vi "Shrug Pipette.vi"(4 "Pressure Controls":T1, 6 "Pressure Levels":refnum<vi>, 8 "error in (no error)":errorcluster, 10 "Manipulator Dynamics":refnum<vi>, 11 "VISA resource in":refnum<visa-resource-name>="COM1") -> (0 "error out":errorcluster, 3 "VISA resource out":refnum<visa-resource-name>)   [LabVIEW 2012, in "Autopatcher Daemon.lvlib"]
uses:
  Autopatcher Daemon.lvlib
  Scientifica Manipulator Controls.lvlib
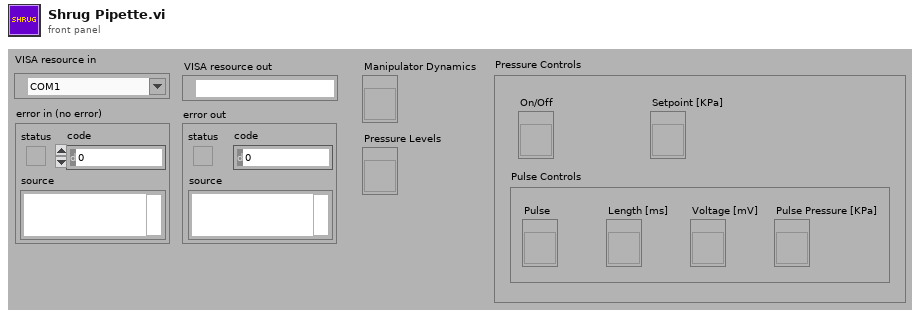
[diagram p1: front panel]
types:
  T1 = cluster{"Setpoint [KPa]":refnum<vi>, "On/Off":refnum<vi>, "Pulse Controls":cluster{"Pulse":refnum<vi>, "Length [ms]":refnum<vi>, "Voltage [mV]":refnum<vi>, "Pulse Pressure [KPa]":refnum<vi>}}
  T2 = cluster{"First Speed [um/s]":i32, "Top Speed [um/s]":i32, "Acceleration [um/s2]":i32, "Step Size [um]":i32, "Interstep Interval [ms]":u32, "Max Depth [um]":i32, "Max Penetration [um]":i32}
  T3 = cluster{"High Pressure Setpoint [KPa]":dbl, "Low Pressure Setpoint [KPa]":dbl, "Min Pressure Setpoint [KPa]":dbl}
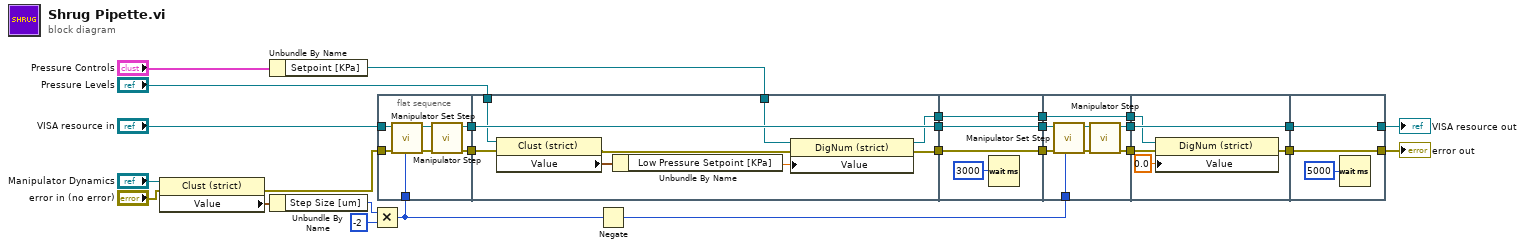
[diagram p0: block diagram]
diagram:
  n1 = property class="Clust (strict)"(reference="Manipulator Dynamics", error in="error in (no error)") -> (error out=w2:errorcluster, "Value"=w9:T2)  [unwired: 1 out]
  n2 = Unbundle By Name("Pressure Controls") -> ("Setpoint [KPa]"=w6:refnum<vi>)
  n3 = Unbundle By Name(w9) -> ("Step Size [um]"=w26:i32)
  n4 = Multiply(x=w26, y=-2 ("x")) -> (x*y=w14:i32)
  n5 = flat-sequence {
    tunnel: w14 -> [w28]
    tunnel: "VISA resource in" -> [w34]
    tunnel: w2 -> [w33]
    tunnel: [w30] -> w24
    tunnel: [w29] -> w21
    tunnel: w24 -> [w43]
    tunnel: [w43] -> w23
    tunnel: w21 -> [w41]
    tunnel: [w37] -> w20
    tunnel: "Pressure Levels" -> [w40]
    tunnel: w6 -> [w36]
    tunnel: [w35] -> w3
    tunnel: w23 -> [w46]
    tunnel: [w46] -> w22
    tunnel: w20 -> [w45]
    tunnel: [w45] -> w19
    tunnel: [w44] -> w4
    tunnel: w3 -> [w44]
    tunnel: w22 -> [w55]
    tunnel: w19 -> [w54]
    tunnel: [w51] -> w16
    tunnel: [w50] -> w15
    tunnel: w13 -> [w49]
    tunnel: [w48] -> w5
    tunnel: w4 -> [w48]
    tunnel: w16 -> [w60]
    tunnel: w15 -> [w59]
    tunnel: [w60] -> w12
    tunnel: [w58] -> w11
    tunnel: w5 -> [w57]
    tunnel: [w62] -> w17
    tunnel: [w63] -> w18
    tunnel: w12 -> [w63]
    tunnel: w11 -> [w62]
    frame #0 {
      n6 = call "Manipulator Set Step.vi"("error in (no error)"=w33, "Step"=w28, "VISA resource in"=w34) -> ("error out"=w32:errorcluster, "VISA resource out"=w31:refnum<visa-resource-name>)  [unwired: 6 in, 1 out]
      n7 = call "Manipulator Step.vi"("error in (no error)"=w32, "VISA resource in"=w31) -> ("error out"=w29:errorcluster, "VISA resource out"=w30:refnum<visa-resource-name>)  [unwired: 7 in, 1 out]
    }
    frame #1 {
      n8 = property class="Clust (strict)"(reference=w40, error in=w41) -> (error out=w39:errorcluster, "Value"=w42:T3)  [unwired: 1 out]
      n9 = Unbundle By Name(w42) -> ("Low Pressure Setpoint [KPa]"=w38:dbl)
      n10 = property class="DigNum (strict)"(reference=w36, error in=w39, "Value"=w38) -> (reference out=w35:refnum<vi>, error out=w37:errorcluster)
    }
    frame #2 {
      n11 = Wait (ms)(milliseconds to wait=u32 3000) -> ()  [unwired: 1 out]
    }
    frame #3 {
      n12 = call "Manipulator Set Step.vi"("error in (no error)"=w54, "Step"=w49, "VISA resource in"=w55) -> ("error out"=w52:errorcluster, "VISA resource out"=w53:refnum<visa-resource-name>)  [unwired: 6 in, 1 out]
      n13 = call "Manipulator Step.vi"("error in (no error)"=w52, "VISA resource in"=w53) -> ("error out"=w50:errorcluster, "VISA resource out"=w51:refnum<visa-resource-name>)  [unwired: 7 in, 1 out]
    }
    frame #4 {
      n14 = property class="DigNum (strict)"(reference=w57, error in=w59, "Value"=0.0) -> (error out=w58:errorcluster)  [unwired: 1 out]
    }
    frame #5 {
      n15 = Wait (ms)(milliseconds to wait=u32 5000) -> ()  [unwired: 1 out]
    }
  }
  n16 = Negate(x=w14) -> (-x=w13:i32)
  "VISA resource out" <- w18
  "error out" <- w17
